vi "On Change Camera Format.vi"(8 "error in (no error)":errorcluster, 10 "Selection":i32, 11 "App in":refnum<class "App.lvclass">) -> (0 "error out":errorcluster, 3 "App out":refnum<class "App.lvclass">)   [LabVIEW 2020, in "AR Example.lvlib" / "App.lvclass"]
uses:
  App.lvclass
  App.lvclass/App.ctl
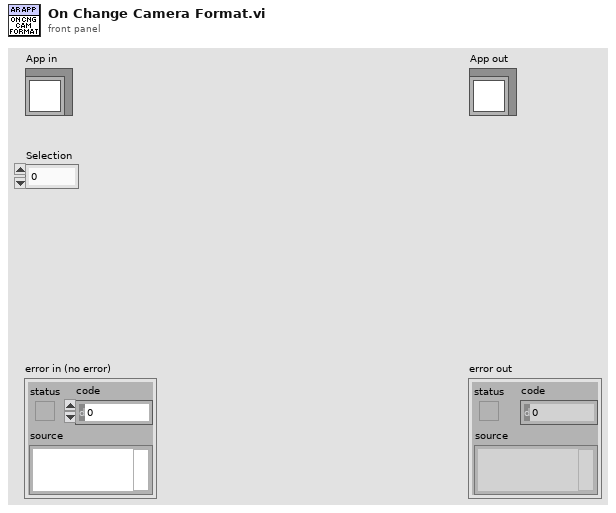
[diagram p1: front panel]
types:
  T1 = typedef "g_ar_toolkit.capture.lvlib/CameraStream.lvclass/Device Enumeration.ctl" = cluster{"Name":string, "Streams":set{T2}}
  T2 = typedef "g_ar_toolkit.capture.lvlib/CameraStream.lvclass/Stream Parameters.ctl" = cluster{"Width":u16, "Height":u16, "FPS":u8}
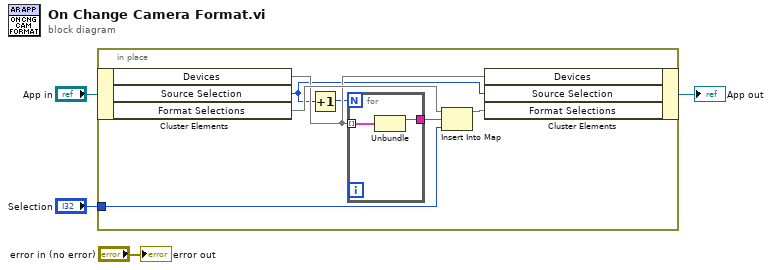
[diagram p0: block diagram]
diagram:
  n1 = in-place {
    in-place-border: "Selection" -> [w9]
    n2 = in-place-cluster #1("App in") -> ("Devices"=w8:map{string, T1}, "Source Selection"=w7:i32, "Format Selections"=w11:map{string, i32})
    n3 = Increment(x=w7) -> (x+1=w5:i32)
    n4 = for {
      N: w5 -> [_]
      tunnel: w8 -> [w13] mode=indexing
      tunnel: [w12] -> w6
      n5 = Unbundle(w13) -> ("id"=w12:string)  [unwired: 1 out]
    }
    n6 = Insert Into Map(map in=w11, key=w6, value=w9) -> (map out=w10:map{string, i32})  [unwired: 2 out]
    n7 = in-place-cluster #1("Devices"=w8, "Source Selection"=w7, "Format Selections"=w10) -> (→"App out":refnum<class "App.lvclass">)
  }
  "error out" <- "error in (no error)"
